vi "Write configuration.vi"(8 "error in (no error)":errorcluster, 11 "Template in":refnum<class "Template.lvclass">) -> (0 "error out":errorcluster, 3 "Template out":refnum<class "Template.lvclass">)   [LabVIEW 2012, in "Template.lvclass"]
doc: "Writes the configuration cluster into the configuration file. Configuration file is XML-based. It's name is <component ID>.xml"
uses:
  Template.lvclass
  <vilib>/Distrio/Murmex/Murmex/Murmex.lvclass
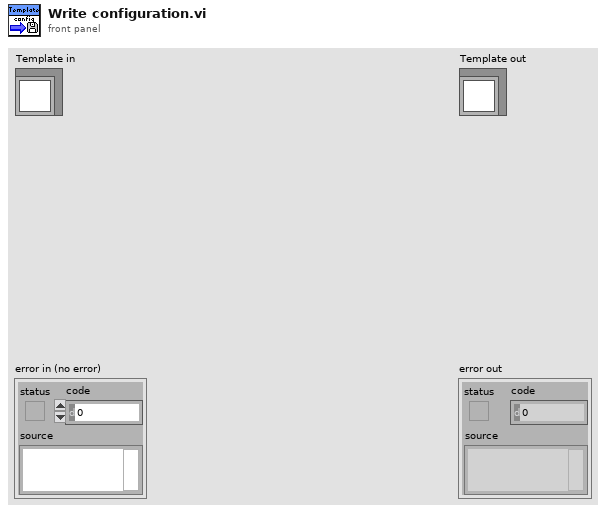
[diagram p1: front panel]
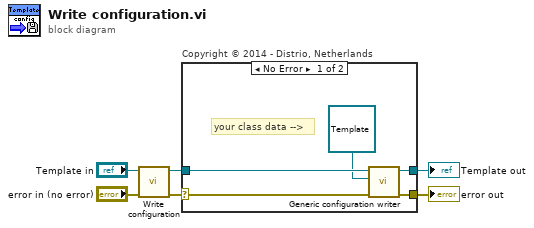
[diagram p0: block diagram]
diagram:
  n1 = call-parent "Write configuration.vi"("error in (no error)"="error in (no error)", "Murmex in"="Template in") -> ("error out"=w4:errorcluster, "Murmex out"=w2:refnum<class "Template.lvclass">)  [unwired: 8 in]
  n2 = case "Copyright © 2014 - Distrio, Netherlands" shown="No Error" w4 {
    selector: w4 -> [w11 w13]
    tunnel: [w10 w13] -> w3
    tunnel: [w8 w12] -> w1
    tunnel: w2 -> [w9 w12]
    frame No Error {
      # "your class data -->"
      n3 = call <vilib>:"Generic configuration writer.vi"("error in (no error)"=w11, "inheritance level"=refnum<class "Template.lvclass"> refnum ("Template.lvclass"), "Murmex in"=w9) -> ("error out"=w10:errorcluster, "Murmex out"=w8:refnum<class "Template.lvclass">)  [unwired: 7 in]
    }
    frame Error {
    }
  }
  "error out" <- w3
  "Template out" <- w1
